vi "SharedVariableServant.vi"() -> ()   [LabVIEW 2014]
uses:
  <vilib>/myRIO/Instrument Drivers/Onboard IO/DIO/typedefs/DIO Reference.ctl
  <vilib>/myRIO/Common/Instrument Driver Framework/Utilities/typedefs/myRIO Generic Hardware Reference.ctl
  <vilib>/myRIO/Common/Instrument Driver Framework/Utilities/typedefs/Hardware Version Enum.ctl
  <vilib>/myRIO/Common/Instrument Driver Framework/Utilities/typedefs/myRIO v1.0 Reference.ctl
  <vilib>/myRIO/Common/Instrument Driver Framework/Utilities/typedefs/Generic FPGA Reference.ctl
  <vilib>/myRIO/Common/Instrument Driver Framework/myRIO v1.0/DIO/typedefs/DIO Channels List.ctl
  <vilib>/myRIO/Common/Instrument Driver Framework/myRIO v1.0/DIO/typedefs/DIO Channels Enum.ctl
  <vilib>/userdefined/High Color/nirio_resource_hc.ctl
  <vilib>/myRIO/Common/Instrument Driver Framework/Utilities/vis/Is FPGA Ref Available.vi
  <vilib>/myRIO/Common/Instrument Driver Framework/myRIO v1.0/DIO/vis/myRIO v1.1 Open DIO.vi
  <vilib>/myRIO/Instrument Drivers/Onboard IO/DIO/vis/Write.vi
  <vilib>/myRIO/Common/Instrument Driver Framework/Utilities/vis/Validate Channels.vi
  <vilib>/myRIO/Common/Instrument Driver Framework/myRIO v1.0/DIO/vis/myRIO v1.0 Reserve DIO.vi
  <vilib>/myRIO/Common/Instrument Driver Framework/myRIO v1.0/UART/vis/myRIO v1.0 Close UART.vi
  <vilib>/myRIO/Common/Instrument Driver Framework/myRIO v1.0/Resource Manager/vis/myRIO v1.0 Reserve Channel List.vi
  <vilib>/myRIO/Common/Instrument Driver Framework/myRIO v1.0/DIO/vis/myRIO v1.0 Build MUX Configuration DIO.vi
  <vilib>/myRIO/Common/Instrument Driver Framework/myRIO v1.0/Resource Manager/vis/myRIO v1.0 Reserve Channel.vi
  <vilib>/myRIO/Common/Instrument Driver Framework/myRIO v1.0/Resource Manager/vis/myRIO v1.0 Unreserve Channel.vi
  <vilib>/myRIO/Common/Instrument Driver Framework/myRIO v1.0/Resource Manager/vis/myRIO v1.0 Create Configuration List.vi
  <vilib>/myRIO/Common/Instrument Driver Framework/myRIO v1.0/Resource Manager/vis/myRIO v1.0 Build Mutex Name.vi
  <vilib>/Utility/VariantDataType/GetNumericInfo.vi
  <vilib>/Utility/error.llb/Error Cluster From Error Code.vi
  <vilib>/myRIO/Common/Instrument Driver Framework/myRIO v1.0/myRIO v1.1 Open.vi
  <vilib>/myRIO/Common/Instrument Driver Framework/Utilities/vis/IO Manager.vi
  <vilib>/myRIO/Common/Instrument Driver Framework/Utilities/vis/Configuration Manager.vi
  <vilib>/myRIO/Common/Instrument Driver Framework/myRIO v1.0/Resource Manager/vis/myRIO v1.0 Configure IO.vi
  <vilib>/myRIO/Common/Instrument Driver Framework/myRIO v1.0/myRIO v1.0 Close.vi
  <vilib>/myRIO/Common/Instrument Driver Framework/myRIO v1.0/DIO/vis/myRIO v1.0 Write DIO.vi
  <vilib>/myRIO/Common/Instrument Driver Framework/Utilities/vis/FPGA Ref Manager.vi
  <vilib>/myRIO/Common/Instrument Driver Framework/myRIO v1.0/myRIO v1.0 Reset FPGA.vi
  <vilib>/myRIO/Common/Instrument Driver Framework/myRIO v1.0/IRQ/vis/myRIO v1.0 IRQ Info FGV.vi
  <vilib>/myRIO/Common/Instrument Driver Framework/myRIO v1.0/IRQ/vis/myRIO v1.0 Timer IRQ Info FGV.vi
  <vilib>/myRIO/Common/Instrument Driver Framework/myRIO v1.0/IRQ/vis/myRIO v1.0 ISR Agent.vi
  <vilib>/myRIO/Express VI/Onboard IO/DO/DO Express VI.xnode
  <vilib>/myRIO/Instrument Drivers/Onboard IO/DIO/vis/myRIO DIO Open.xnode
  <vilib>/myRIO/Instrument Drivers/Utilities/Utilities.lvlib
  <vilib>/myRIO/Instrument Drivers/Onboard IO/DIO/DIO.lvlib
panel:
  in  "Outlet5_Refnum":refnum<k21>="ni.var.psp://Deepak-PC/Shared Variable Library Master/Outlet5"
  in  "Outlet4_Refnum":refnum<k21>="ni.var.psp://Deepak-PC/Shared Variable Library Master/Outlet4"
  in  "Outlet3_Refnum":refnum<k21>="ni.var.psp://Deepak-PC/Shared Variable Library Master/Outlet3"
  in  "Outlet2_Refnum":refnum<k21>="ni.var.psp://Deepak-PC/Shared Variable Library Master/Outlet2"
  in  "Outlet1_Refnum":refnum<k21>="ni.var.psp://Deepak-PC/Shared Variable Library Master/Outlet1"
  in  "Stop":bool
  out "Outlet1_Output":bool
  out "Outlet2_Output":bool
  out "Outlet3_Output":bool
  out "Outlet4_Output":bool
  out "Outlet5_Output":bool
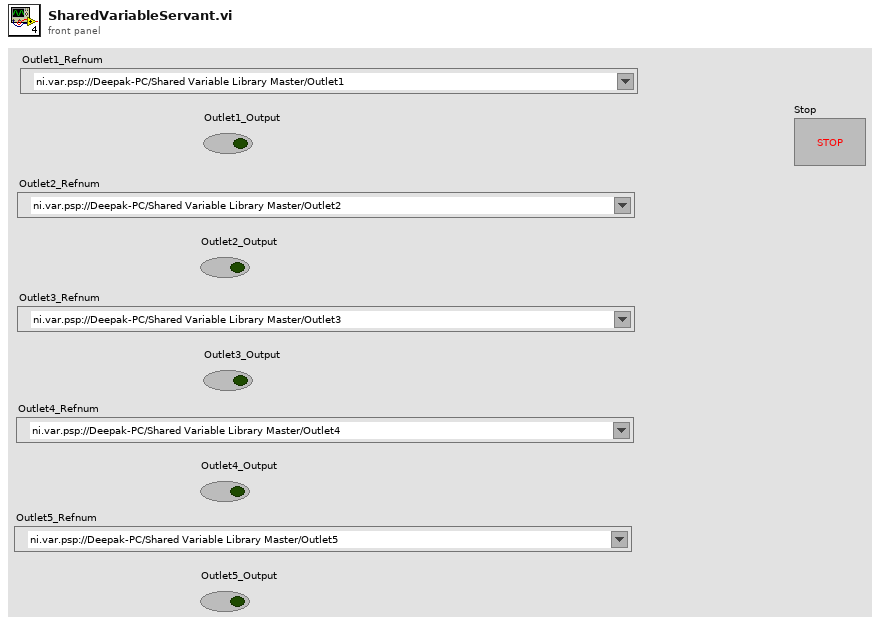
[diagram p1: front panel]
types:
  T1 = typedef "DIO.lvlib/DIO Reference.ctl" = cluster{"myRIO Reference":T2, "DIO Channels List":T6}
  T2 = typedef "myRIO Generic Hardware Reference.ctl" = cluster{"myRIO Model":T3, "myRIO Hardware Reference":T4}
  T3 = typedef "Hardware Version Enum.ctl" = enum16{"Unknown", "myRIO-1900", "myRIO-1950"}
  T4 = typedef "myRIO v1.0 Reference.ctl" = cluster{"Generic FPGA Reference":T5, "Allow multiple opens":bool}
  T5 = typedef "Generic FPGA Reference.ctl" = refnum<k20>
  T6 = typedef "DIO Channels List.ctl" = T7[]
  T7 = typedef "DIO Channels Enum.ctl" = enum16{"Not Connected", "C/DIO0", "C/DIO1", "C/DIO2", "C/DIO3", "C/DIO4", "C/DIO5", "C/DIO6", "C/DIO7", "A/DIO0", "A/DIO1", "A/DIO2", "A/DIO3", "A/DIO4", "A/DIO5", "A/DIO6", "A/DIO7", "A/DIO8", "A/DIO9", "A/DIO10", "A/DIO11", "A/DIO12", "A/DIO13", "A/DIO14", "A/DIO15", "B/DIO0", "B/DIO1", "B/DIO2", "B/DIO3", "B/DIO4", "B/DIO5", "B/DIO6", "B/DIO7", "B/DIO8", "B/DIO9", "B/DIO10", "B/DIO11", "B/DIO12", "B/DIO13", "B/DIO14", "B/DIO15", "LED0", "LED1", "LED2", "LED3", "Button0"}
  T8 = typedef "nirio_resource_hc.ctl" = tag
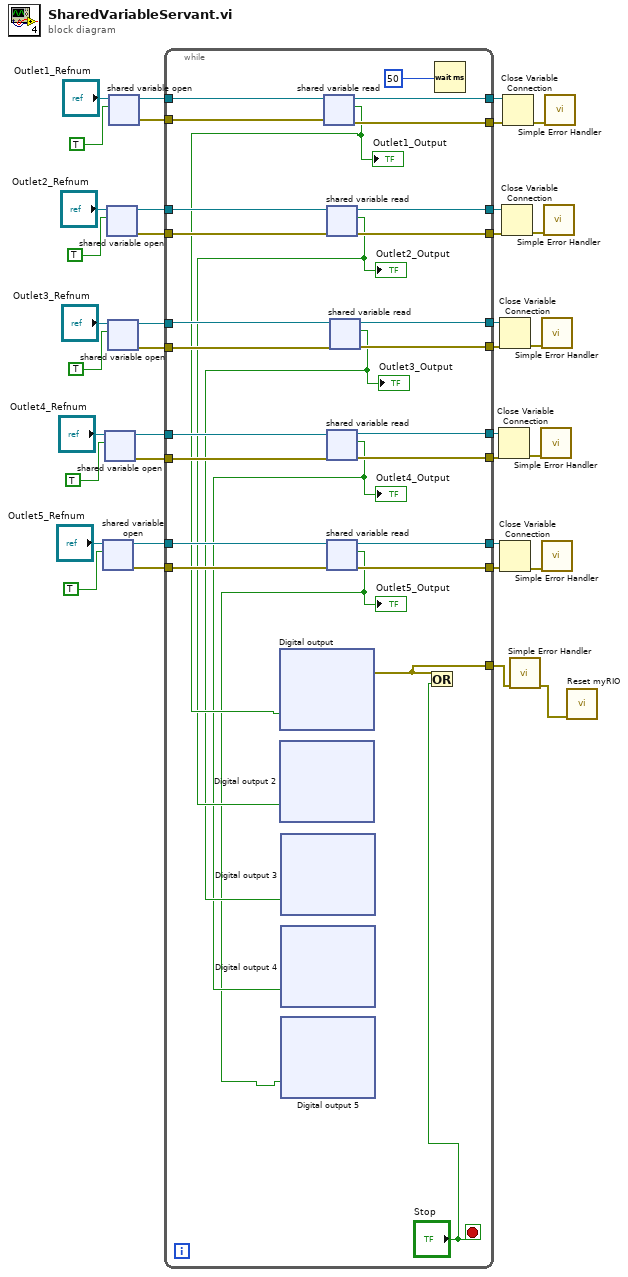
[diagram p0: block diagram]
diagram:
  n1 = shared-variable-open("Outlet5_Refnum", TRUE) -> (w6:refnum<k21>, w4:errorcluster)  [unwired: 2 in]
  n2 = shared-variable-open("Outlet4_Refnum", TRUE) -> (w10:refnum<k21>, w9:errorcluster)  [unwired: 2 in]
  n3 = shared-variable-open("Outlet2_Refnum", TRUE) -> (w27:refnum<k21>, w26:errorcluster)  [unwired: 2 in]
  n4 = shared-variable-open("Outlet3_Refnum", TRUE) -> (w14:refnum<k21>, w13:errorcluster)  [unwired: 2 in]
  n5 = shared-variable-open("Outlet1_Refnum", TRUE) -> (w34:refnum<k21>, w33:errorcluster)  [unwired: 2 in]
  n6 = while {
    tunnel: w34 -> [w54]
    tunnel: w33 -> [w53]
    tunnel: [w64] -> w32
    tunnel: [w63] -> w31
    tunnel: w27 -> [w52]
    tunnel: w26 -> [w51]
    tunnel: [w62] -> w25
    tunnel: [w61] -> w24
    tunnel: w14 -> [w50]
    tunnel: w13 -> [w49]
    tunnel: [w60] -> w12
    tunnel: [w59] -> w11
    tunnel: w10 -> [w48]
    tunnel: w9 -> [w47]
    tunnel: [w58] -> w8
    tunnel: [w57] -> w7
    tunnel: w6 -> [w46]
    tunnel: [w56] -> w5
    tunnel: w4 -> [w45]
    tunnel: [w55] -> w3
    tunnel: [w43] -> w1
    stop <- "Stop" stop-if-true
    n7 = shared-variable-read(w54, w53) -> (w64:refnum<k21>, w63:errorcluster, w42:bool)  [unwired: 1 out]
    "Outlet1_Output" <- w42
    n8 = xnode "Digital output"("B/DIO0 (Pin 11)"=w42) -> ("error out"=w43:errorcluster)  [unwired: 1 in]
    n9 = shared-variable-read(w52, w51) -> (w62:refnum<k21>, w61:errorcluster, w41:bool)  [unwired: 1 out]
    "Outlet2_Output" <- w41
    n10 = xnode "Digital output 2"("A/DIO1 (Pin 13)"=w41) -> ()  [unwired: 1 in, 1 out]
    n11 = shared-variable-read(w48, w47) -> (w58:refnum<k21>, w57:errorcluster, w39:bool)  [unwired: 1 out]
    "Outlet4_Output" <- w39
    n12 = xnode "Digital output 4"("B/DIO3 (Pin 17)"=w39) -> ()  [unwired: 1 in, 1 out]
    n13 = shared-variable-read(w46, w45) -> (w56:refnum<k21>, w55:errorcluster, w38:bool)  [unwired: 1 out]
    "Outlet5_Output" <- w38
    n14 = xnode "Digital output 5"("B/DIO4 (Pin 19)"=w38) -> ()  [unwired: 1 in, 1 out]
    n15 = shared-variable-read(w50, w49) -> (w60:refnum<k21>, w59:errorcluster, w40:bool)  [unwired: 1 out]
    "Outlet3_Output" <- w40
    n16 = xnode "Digital output 3"("B/DIO2 (Pin 15)"=w40) -> ()  [unwired: 1 in, 1 out]
    n17 = Or(x=w43, y="Stop") -> ()  [unwired: 1 out]
    n18 = Wait (ms)(milliseconds to wait=u32 50 ("millisecond timer value")) -> ()  [unwired: 1 out]
  }
  n19 = Close Variable Connection(8:w7, 11:w8) -> (0:w17:errorcluster)
  n20 = Close Variable Connection(8:w11, 11:w12) -> (0:w16:errorcluster)
  n21 = Close Variable Connection(8:w3, 11:w5) -> (0:w15:errorcluster)
  n22 = Close Variable Connection(8:w24, 11:w25) -> (0:w28:errorcluster)
  n23 = Close Variable Connection(8:w31, 11:w32) -> (0:w35:errorcluster)
  n24 = call <vilib>:"Simple Error Handler.vi"("error in (no error)"=w1) -> ("error out"=w2:errorcluster)  [unwired: 4 in, 4 out]
  n25 = call <vilib>:"Simple Error Handler.vi"("error in (no error)"=w17) -> ()  [unwired: 4 in, 5 out]
  n26 = call <vilib>:"Simple Error Handler.vi"("error in (no error)"=w16) -> ()  [unwired: 4 in, 5 out]
  n27 = call <vilib>:"Simple Error Handler.vi"("error in (no error)"=w15) -> ()  [unwired: 4 in, 5 out]
  n28 = call <vilib>:"Simple Error Handler.vi"("error in (no error)"=w28) -> ()  [unwired: 4 in, 5 out]
  n29 = call <vilib>:"Simple Error Handler.vi"("error in (no error)"=w35) -> ()  [unwired: 4 in, 5 out]
  n30 = call <vilib>:"Reset myRIO.vi"("error in (no error)"=w2) -> ()  [unwired: 10 in, 1 out]
